vi "Read OPC ALRName.vi"(8 "error in (no error)":errorcluster, 11 "Refnum in":T1) -> (0 "error out":errorcluster, 3 "values":string[](array[string]))   [LabVIEW 2019, in "OPC addons.lvlib"]
uses:
  OPC addons.lvlib
  <vilib>/OPCUA/controls/OPC UA Client Refnum.ctl
  <vilib>/OPCUA/controls/NodeIds.ctl
  <vilib>/OPCUA/controls/NodeId.ctl
  <vilib>/OPCUA/client/Multiple Read String Array.vi
  <vilib>/OPCUA/NI OPC UA Client.lvlib
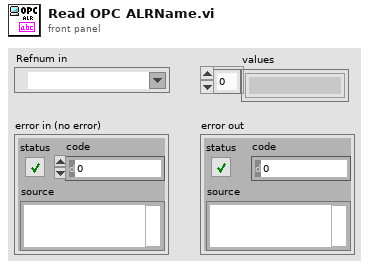
[diagram p1: front panel]
types:
  T1 = typedef "OPC UA Client Refnum.ctl" = refnum<k21>
  T2 = typedef "NodeIds.ctl" = T3[]
  T3 = typedef "NodeId.ctl" = string
  T4 = typedef "OPC UA StatusCode.ctl" = u32
  T5 = cluster{"node ID":T3, "values ":string[], "timestamp":timestamp, "status":T4}[]
  T6 = cluster{"node ID":T3, "values ":string[], "timestamp":timestamp, "status":T4}
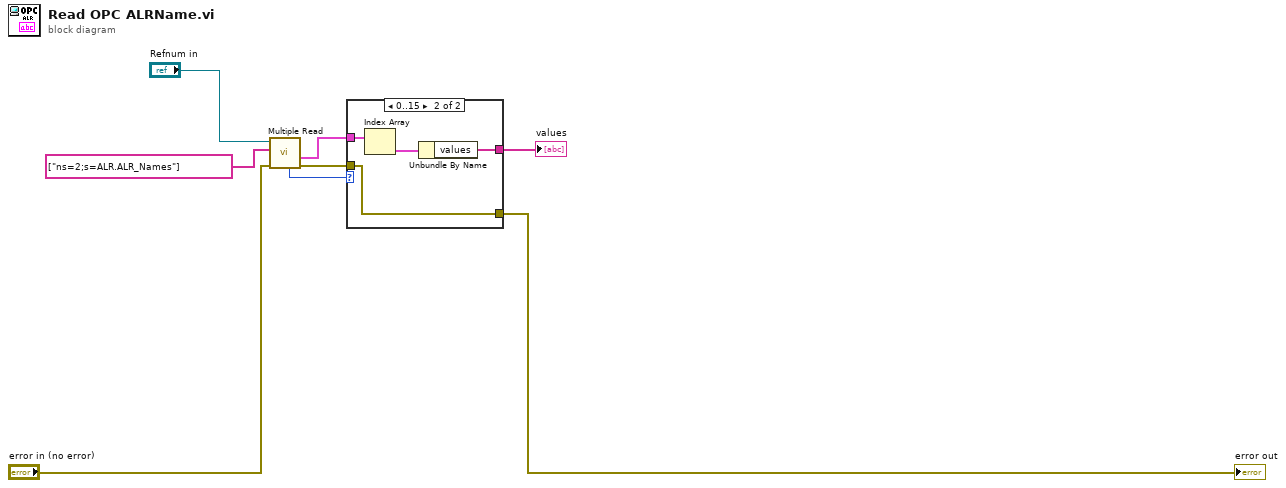
[diagram p0: block diagram]
diagram:
  n1 = call-poly <vilib>:"Multiple Read.vi"("error in (no error)"="error in (no error)", "node IDs"=T2 ["ns=2;s=ALR.ALR_Names"] ("OPC UA.node IDs"), "OPC UA client refnum in"="Refnum in") -> ("error out"=w2:errorcluster, "results"=w1:T5, "service status"=w3:T4)  [unwired: 5 in, 1 out]
  n2 = case shown="0..15" w3 {
    tunnel: w2 -> [w9 w10]
    tunnel: [w9 w10] -> w6
    tunnel: w1 -> [_ w12]
    tunnel: [_ w11] -> w8
    frame 16.., Default {
    }
    frame 0..15 {
      n3 = Index Array(array=w12) -> (element=w13:T6)  [unwired: 1 in]
      n4 = Unbundle By Name(w13) -> ("values"=w11:string[])
    }
  }
  "values" <- w8
  "error out" <- w6
